vi "Set Panel Origin.vi"(8 "error in":errorcluster, 11 "VI Ref In":refnum<vi>) -> (0 "error out":errorcluster, 3 "VI Ref Out":refnum<vi>)   [LabVIEW 2023]
doc: "Scroll all panes on referenced VI (defaults to parent VI if not wired) to pane orgin."
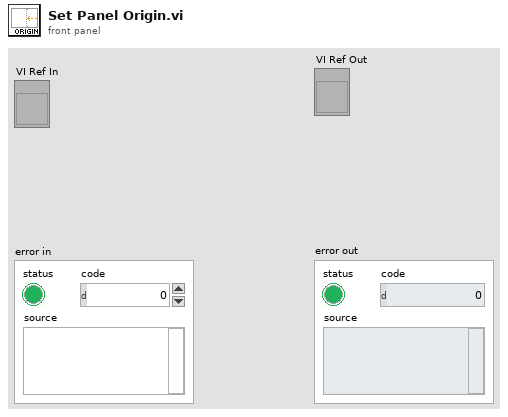
[diagram p1: front panel]
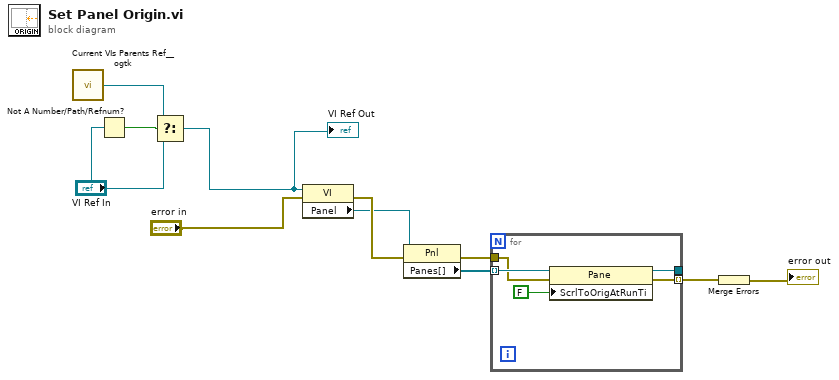
[diagram p0: block diagram]
diagram:
  n1 = call <userlib>:"Current VIs Parents Ref__ogtk.vi"() -> ("Calling VI's Reference"=w6:refnum<vi>)  [unwired: 2 in]
  n2 = Not A Number/Path/Refnum?(number/path/refnum="VI Ref In") -> (NaN/Path/Refnum?=w7:bool)
  n3 = Select(t=w6, s=w7, f="VI Ref In") -> (s? t:f=w4:refnum<vi>)
  "VI Ref Out" <- w4
  n4 = property class="VI"(reference=w4, error in="error in") -> (error out=w10:errorcluster, "Panel"=w8:refnum<vi>)  [unwired: 1 out]
  n5 = property class="Pnl"(reference=w8, error in=w10) -> (error out=w9:errorcluster, "Panes[]"=w11:refnum<vi>[])  [unwired: 1 out]
  n6 = for {
    tunnel: w11 -> [w16] mode=indexing
    tunnel: [w15] -> _
    tunnel: w9 -> [w14]
    tunnel: [w13] -> w3 mode=indexing
    n7 = property class="Pane"(reference=w16, error in=w14, "ScrlToOrigAtRunTi"=FALSE ("Scroll To Origin At Run Time")) -> (reference out=w15:refnum<vi>, error out=w13:errorcluster)
  }
  n8 = Merge Errors(w3) -> (→"error out":errorcluster)
